vi "ordersCH3.vi"(8 "错误输入（无错误）":errorcluster, 9 "关闭通道":u16(ring)=1 items=["CH1", "CH2", "CH3", "CH4"], 10 "打开通道":u16(ring)=2 items=["CH1", "CH2", "CH3", "CH4"], 11 "VISA资源名称":refnum<visa-resource-name>="DPO5054-C012667") -> (0 "错误输出":errorcluster, 2 "输出数组":dbl[](array[numeric]))   [LabVIEW 2014]
panel:
  out "AMP":dbl
  out "RMS":dbl
  out "MAX":dbl
  out "MIN":dbl
  out "PK2PK":dbl
  out "PERIOD":dbl
  out "FREQ":dbl
  out "RISETIME":dbl
  out "FallTime":dbl
  out "PosWidth":dbl
  out "NegWidth":dbl
  out "PositiveDutyCycle":dbl
  out "NegativeDutyCycle":dbl
  out "ACRMS":dbl
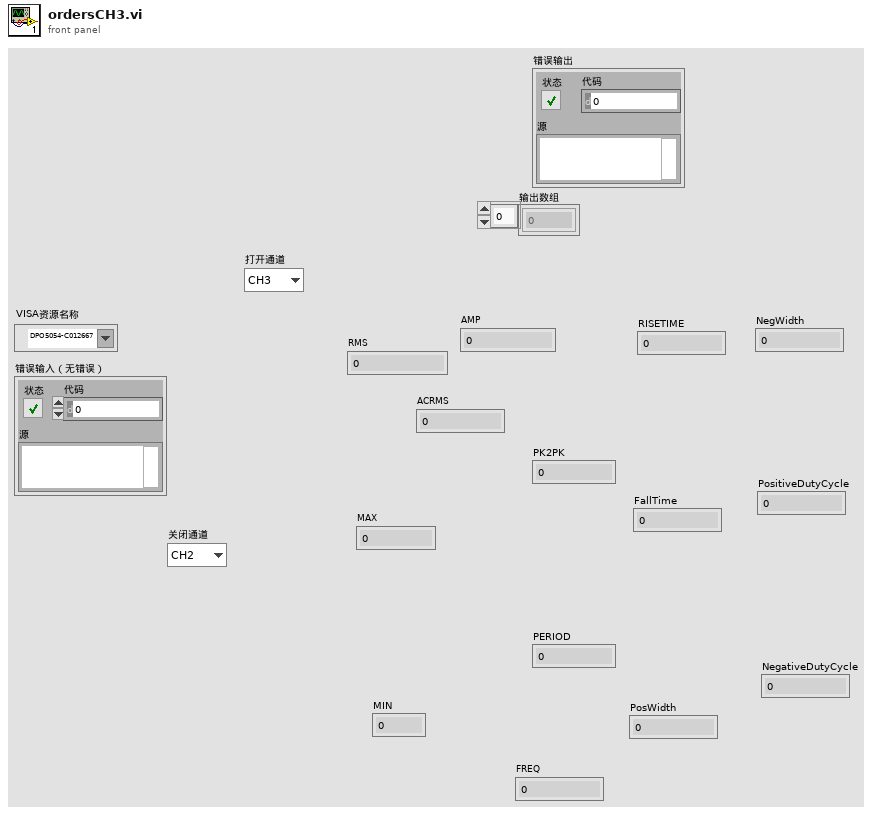
[diagram p1: front panel]
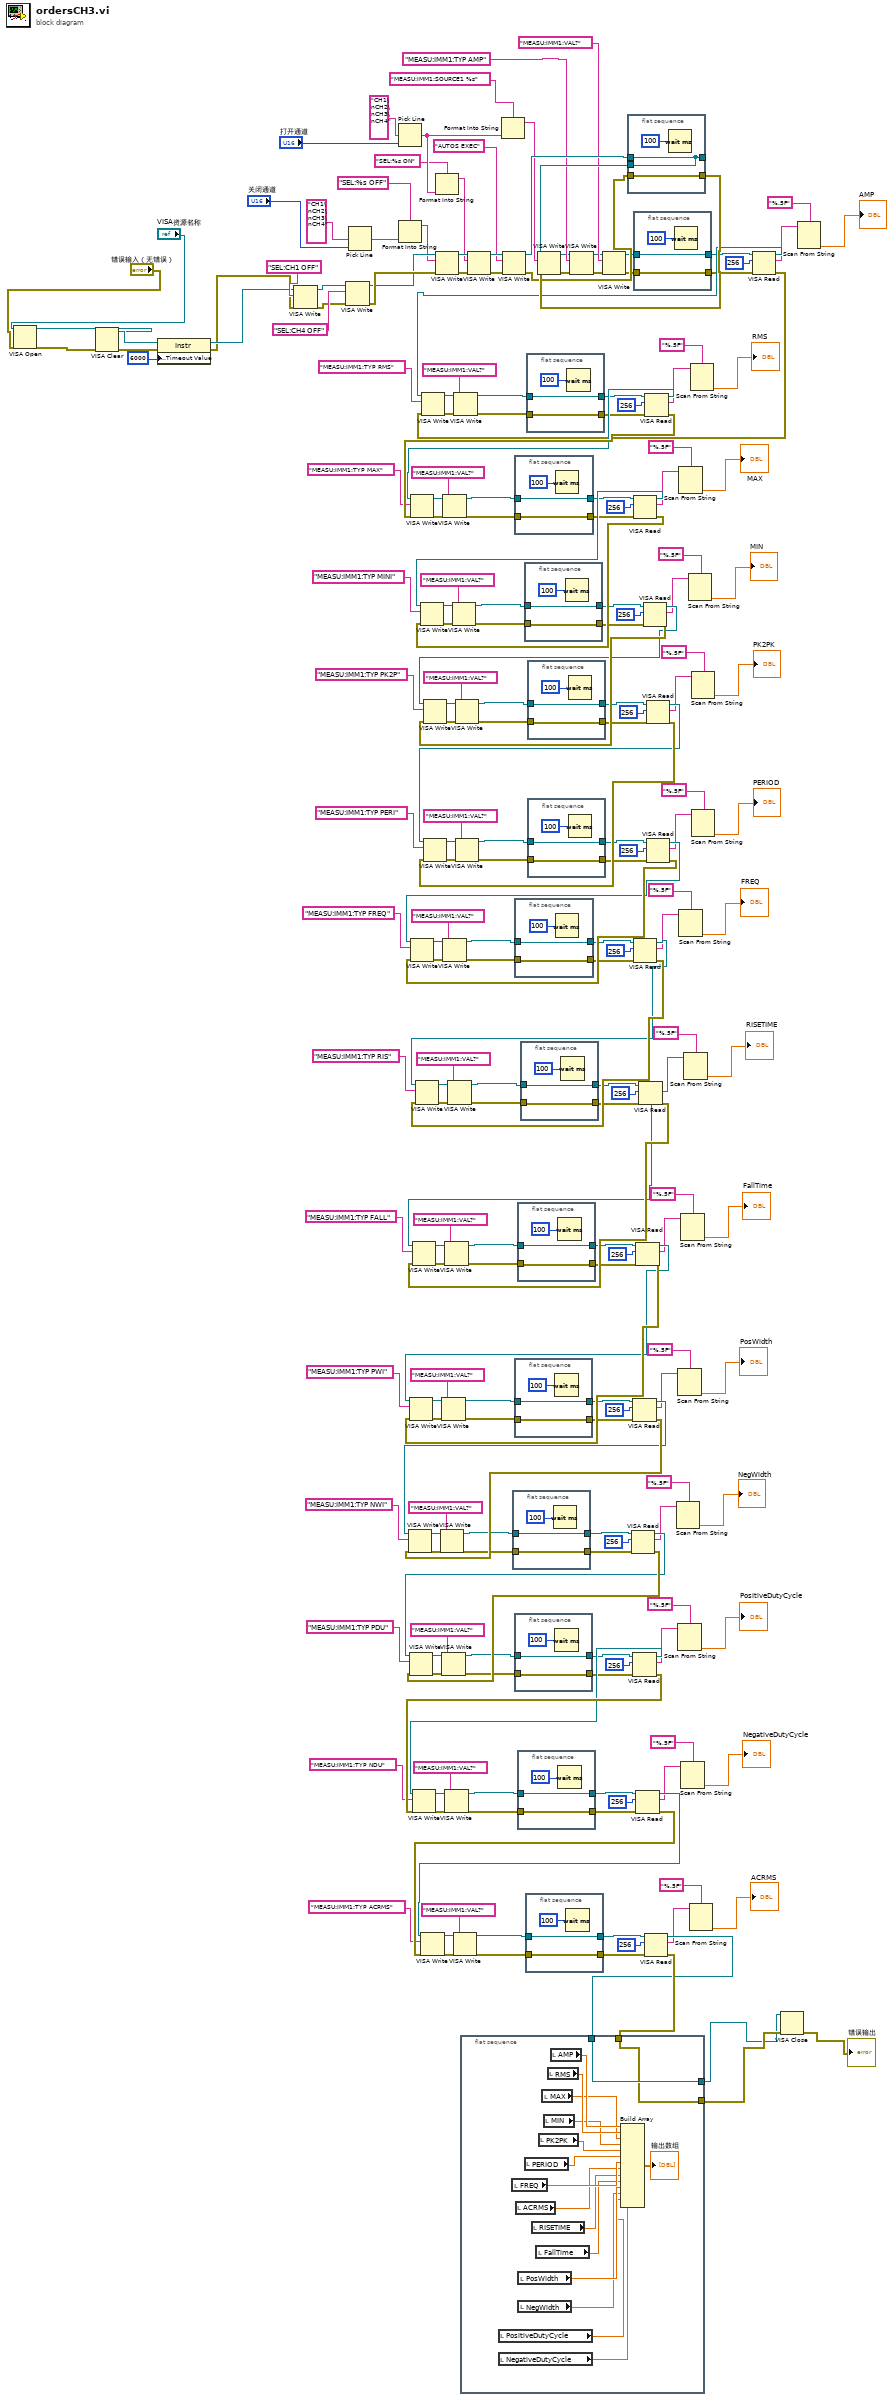
[diagram p0: block diagram]
diagram:
  n1 = VISA Open(error in (no error)="错误输入（无错误）", VISA resource name="VISA资源名称") -> (VISA resource name=w221:refnum<visa-resource-name>, error out=w222:errorcluster)  [unwired: 3 in]
  n2 = VISA Clear(VISA resource name=w221, error in (no error)=w222) -> (VISA resource name out=w223:refnum<visa-resource-name>, error out=w224:errorcluster)
  n3 = property class="Instr"(reference=w223, error in=w224, "General Settings:Timeout Value"=u32 6000) -> (reference out=w231:refnum<visa-resource-name>, error out=w230:errorcluster)
  n4 = VISA Write(VISA resource name=w231, write buffer="SEL:CH1 OFF" ("格式字符串"), error in (no error)=w230) -> (VISA resource name out=w233:refnum<visa-resource-name>, error out=w234:errorcluster)  [unwired: 1 out]
  n5 = VISA Write(VISA resource name=w233, write buffer="SEL:CH4 OFF" ("格式字符串"), error in (no error)=w234) -> (VISA resource name out=w236:refnum<visa-resource-name>, error out=w237:errorcluster)  [unwired: 1 out]
  n6 = Pick Line(multi-line string="CH1\nCH2\nCH3\nCH4" ("多行字符串"), line index="关闭通道") -> (output string=w21:string)  [unwired: 1 in]
  n7 = Pick Line(multi-line string="CH1\nCH2\nCH3\nCH4" ("多行字符串"), line index="打开通道") -> (output string=w16:string)  [unwired: 1 in]
  n8 = Format Into String(format string="SEL:%s OFF" ("格式字符串"), w21) -> (resulting string=w25:string)  [unwired: 2 in, 1 out]
  n9 = Format Into String(format string="SEL:%s ON" ("格式字符串"), w16) -> (resulting string=w17:string)  [unwired: 2 in, 1 out]
  n10 = VISA Write(VISA resource name=w236, write buffer=w25, error in (no error)=w237) -> (VISA resource name out=w26:refnum<visa-resource-name>, error out=w27:errorcluster)  [unwired: 1 out]
  n11 = flat-sequence {
    tunnel: w218 -> [w239]
    tunnel: [w239] -> w227
    tunnel: w219 -> [w238]
    tunnel: [w238] -> w228
    frame #0 {
      n12 = local read "PositiveDutyCycle"() -> (w242:dbl)
      n13 = local read "NegativeDutyCycle"() -> (w241:dbl)
      n14 = local read "FREQ"() -> (w248:dbl)
      n15 = local read "ACRMS"() -> (w247:dbl)
      n16 = local read "PosWidth"() -> (w244:dbl)
      n17 = local read "NegWidth"() -> (w243:dbl)
      n18 = local read "PERIOD"() -> (w249:dbl)
      n19 = local read "RISETIME"() -> (w246:dbl)
      n20 = local read "FallTime"() -> (w245:dbl)
      n21 = local read "PK2PK"() -> (w250:dbl)
      n22 = local read "MAX"() -> (w252:dbl)
      n23 = local read "MIN"() -> (w251:dbl)
      n24 = local read "RMS"() -> (w253:dbl)
      n25 = local read "AMP"() -> (w254:dbl)
      n26 = Build Array(w254, w253, w252, w251, w250, w249, w248, w247, w246, w245, w244, w243, w242, w241) -> (→"输出数组":dbl[])
    }
  }
  n27 = VISA Write(VISA resource name=w26, write buffer=w17, error in (no error)=w27) -> (VISA resource name out=w19:refnum<visa-resource-name>, error out=w20:errorcluster)  [unwired: 1 out]
  n28 = Format Into String(format string="MEASU:IMM1:SOURCE1 %s" ("格式字符串"), w16) -> (resulting string=w3:string)  [unwired: 2 in, 1 out]
  n29 = VISA Write(VISA resource name=w19, write buffer="AUTOS EXEC" ("写入缓冲区"), error in (no error)=w20) -> (VISA resource name out=w116:refnum<visa-resource-name>, error out=w117:errorcluster)  [unwired: 1 out]
  n30 = flat-sequence {
    tunnel: w157 -> [w256]
    tunnel: [w256] -> w159
    tunnel: w156 -> [w255]
    tunnel: [w255] -> w160
    frame #0 {
      n31 = Wait (ms)(milliseconds to wait=u32 100 ("等待时间（毫秒）")) -> ()  [unwired: 1 out]
    }
  }
  n32 = flat-sequence {
    tunnel: w154 -> [w259]
    tunnel: [w259] -> w152
    tunnel: w155 -> [w258]
    tunnel: [w258] -> w151
    frame #0 {
      n33 = Wait (ms)(milliseconds to wait=u32 100 ("等待时间（毫秒）")) -> ()  [unwired: 1 out]
    }
  }
  n34 = flat-sequence {
    tunnel: w178 -> [w262]
    tunnel: [w262] -> w176
    tunnel: w179 -> [w261]
    tunnel: [w261] -> w175
    frame #0 {
      n35 = Wait (ms)(milliseconds to wait=u32 100 ("等待时间（毫秒）")) -> ()  [unwired: 1 out]
    }
  }
  n36 = flat-sequence {
    tunnel: w45 -> [w265]
    tunnel: [w265] -> w47
    tunnel: w44 -> [w264]
    tunnel: [w264] -> w48
    frame #0 {
      n37 = Wait (ms)(milliseconds to wait=u32 100 ("等待时间（毫秒）")) -> ()  [unwired: 1 out]
    }
  }
  n38 = flat-sequence {
    tunnel: w93 -> [w268]
    tunnel: [w268] -> w95
    tunnel: w92 -> [w267]
    tunnel: [w267] -> w96
    frame #0 {
      n39 = Wait (ms)(milliseconds to wait=u32 100 ("等待时间（毫秒）")) -> ()  [unwired: 1 out]
    }
  }
  n40 = flat-sequence {
    tunnel: w133 -> [w271]
    tunnel: [w271] -> w135
    tunnel: w132 -> [w270]
    tunnel: [w270] -> w136
    frame #0 {
      n41 = Wait (ms)(milliseconds to wait=u32 100 ("等待时间（毫秒）")) -> ()  [unwired: 1 out]
    }
  }
  n42 = flat-sequence {
    tunnel: w181 -> [w274]
    tunnel: [w274] -> w183
    tunnel: w180 -> [w273]
    tunnel: [w273] -> w184
    frame #0 {
      n43 = Wait (ms)(milliseconds to wait=u32 100 ("等待时间（毫秒）")) -> ()  [unwired: 1 out]
    }
  }
  n44 = flat-sequence {
    tunnel: w130 -> [w277]
    tunnel: [w277] -> w128
    tunnel: w131 -> [w276]
    tunnel: [w276] -> w127
    frame #0 {
      n45 = Wait (ms)(milliseconds to wait=u32 100 ("等待时间（毫秒）")) -> ()  [unwired: 1 out]
    }
  }
  n46 = flat-sequence {
    tunnel: w66 -> [w280]
    tunnel: [w280] -> w64
    tunnel: w67 -> [w279]
    tunnel: [w279] -> w63
    frame #0 {
      n47 = Wait (ms)(milliseconds to wait=u32 100 ("等待时间（毫秒）")) -> ()  [unwired: 1 out]
    }
  }
  n48 = flat-sequence {
    tunnel: w214 -> [w283]
    tunnel: [w283] -> w212
    tunnel: w215 -> [w282]
    tunnel: [w282] -> w211
    frame #0 {
      n49 = Wait (ms)(milliseconds to wait=u32 100 ("等待时间（毫秒）")) -> ()  [unwired: 1 out]
    }
  }
  n50 = flat-sequence {
    tunnel: w42 -> [w286]
    tunnel: [w286] -> w40
    tunnel: w43 -> [w285]
    tunnel: [w285] -> w39
    frame #0 {
      n51 = Wait (ms)(milliseconds to wait=u32 100 ("等待时间（毫秒）")) -> ()  [unwired: 1 out]
    }
  }
  n52 = flat-sequence {
    tunnel: w69 -> [w289]
    tunnel: [w289] -> w71
    tunnel: w68 -> [w288]
    tunnel: [w288] -> w72
    frame #0 {
      n53 = Wait (ms)(milliseconds to wait=u32 100 ("等待时间（毫秒）")) -> ()  [unwired: 1 out]
    }
  }
  n54 = flat-sequence {
    tunnel: w90 -> [w292]
    tunnel: [w292] -> w88
    tunnel: w91 -> [w291]
    tunnel: [w291] -> w87
    frame #0 {
      n55 = Wait (ms)(milliseconds to wait=u32 100 ("等待时间（毫秒）")) -> ()  [unwired: 1 out]
    }
  }
  n56 = VISA Write(VISA resource name=w118, write buffer=w3, error in (no error)=w119) -> (VISA resource name out=w6:refnum<visa-resource-name>, error out=w7:errorcluster)  [unwired: 1 out]
  n57 = VISA Write(VISA resource name=w6, write buffer="MEASU:IMM1:TYP AMP" ("写入缓冲区"), error in (no error)=w7) -> (VISA resource name out=w10:refnum<visa-resource-name>, error out=w11:errorcluster)  [unwired: 1 out]
  n58 = VISA Write(VISA resource name=w10, write buffer="MEASU:IMM1:VAL?" ("写入缓冲区"), error in (no error)=w11) -> (VISA resource name out=w13:refnum<visa-resource-name>, error out=w14:errorcluster)  [unwired: 1 out]
  n59 = flat-sequence {
    tunnel: w116 -> [w294]
    tunnel: [w294] -> _
    tunnel: w117 -> [w295]
    tunnel: [w295] -> w119
    tunnel: [w294] -> w118
    frame #0 {
      n60 = Wait (ms)(milliseconds to wait=u32 100 ("等待时间（毫秒）")) -> ()  [unwired: 1 out]
    }
  }
  n61 = VISA Read(VISA resource name=w159, byte count=u32 256 ("字节总数"), error in (no error)=w160) -> (VISA resource name out=w200:refnum<visa-resource-name>, read buffer=w161:string, error out=w201:errorcluster)  [unwired: 1 out]
  n62 = VISA Write(VISA resource name=w200, write buffer="MEASU:IMM1:TYP PDU" ("写入缓冲区"), error in (no error)=w201) -> (VISA resource name out=w170:refnum<visa-resource-name>, error out=w169:errorcluster)  [unwired: 1 out]
  n63 = VISA Write(VISA resource name=w170, write buffer="MEASU:IMM1:VAL?" ("写入缓冲区"), error in (no error)=w169) -> (VISA resource name out=w178:refnum<visa-resource-name>, error out=w179:errorcluster)  [unwired: 1 out]
  n64 = VISA Read(VISA resource name=w152, byte count=u32 256 ("字节总数"), error in (no error)=w151) -> (VISA resource name out=w198:refnum<visa-resource-name>, read buffer=w150:string, error out=w199:errorcluster)  [unwired: 1 out]
  n65 = VISA Write(VISA resource name=w198, write buffer="MEASU:IMM1:TYP NWI" ("写入缓冲区"), error in (no error)=w199) -> (VISA resource name out=w165:refnum<visa-resource-name>, error out=w166:errorcluster)  [unwired: 1 out]
  n66 = VISA Write(VISA resource name=w165, write buffer="MEASU:IMM1:VAL?" ("写入缓冲区"), error in (no error)=w166) -> (VISA resource name out=w157:refnum<visa-resource-name>, error out=w156:errorcluster)  [unwired: 1 out]
  n67 = VISA Read(VISA resource name=w176, byte count=u32 256 ("字节总数"), error in (no error)=w175) -> (VISA resource name out=w202:refnum<visa-resource-name>, read buffer=w174:string, error out=w203:errorcluster)  [unwired: 1 out]
  n68 = VISA Write(VISA resource name=w202, write buffer="MEASU:IMM1:TYP NDU" ("写入缓冲区"), error in (no error)=w203) -> (VISA resource name out=w189:refnum<visa-resource-name>, error out=w190:errorcluster)  [unwired: 1 out]
  n69 = VISA Write(VISA resource name=w189, write buffer="MEASU:IMM1:VAL?" ("写入缓冲区"), error in (no error)=w190) -> (VISA resource name out=w181:refnum<visa-resource-name>, error out=w180:errorcluster)  [unwired: 1 out]
  n70 = flat-sequence {
    tunnel: w13 -> [w298]
    tunnel: [w298] -> w8
    tunnel: w14 -> [w297]
    tunnel: [w297] -> w9
    frame #0 {
      n71 = Wait (ms)(milliseconds to wait=u32 100 ("等待时间（毫秒）")) -> ()  [unwired: 1 out]
    }
  }
  n72 = VISA Read(VISA resource name=w47, byte count=u32 256 ("字节总数"), error in (no error)=w48) -> (VISA resource name out=w108:refnum<visa-resource-name>, read buffer=w49:string, error out=w109:errorcluster)  [unwired: 1 out]
  n73 = VISA Write(VISA resource name=w108, write buffer="MEASU:IMM1:TYP MINI" ("写入缓冲区"), error in (no error)=w109) -> (VISA resource name out=w58:refnum<visa-resource-name>, error out=w57:errorcluster)  [unwired: 1 out]
  n74 = VISA Write(VISA resource name=w58, write buffer="MEASU:IMM1:VAL?" ("写入缓冲区"), error in (no error)=w57) -> (VISA resource name out=w66:refnum<visa-resource-name>, error out=w67:errorcluster)  [unwired: 1 out]
  n75 = VISA Read(VISA resource name=w95, byte count=u32 256 ("字节总数"), error in (no error)=w96) -> (VISA resource name out=w192:refnum<visa-resource-name>, read buffer=w97:string, error out=w193:errorcluster)  [unwired: 1 out]
  n76 = VISA Write(VISA resource name=w192, write buffer="MEASU:IMM1:TYP RIS" ("写入缓冲区"), error in (no error)=w193) -> (VISA resource name out=w122:refnum<visa-resource-name>, error out=w121:errorcluster)  [unwired: 1 out]
  n77 = VISA Write(VISA resource name=w122, write buffer="MEASU:IMM1:VAL?" ("写入缓冲区"), error in (no error)=w121) -> (VISA resource name out=w130:refnum<visa-resource-name>, error out=w131:errorcluster)  [unwired: 1 out]
  n78 = VISA Read(VISA resource name=w135, byte count=u32 256 ("字节总数"), error in (no error)=w136) -> (VISA resource name out=w196:refnum<visa-resource-name>, read buffer=w137:string, error out=w197:errorcluster)  [unwired: 1 out]
  n79 = VISA Write(VISA resource name=w196, write buffer="MEASU:IMM1:TYP PWI" ("写入缓冲区"), error in (no error)=w197) -> (VISA resource name out=w146:refnum<visa-resource-name>, error out=w145:errorcluster)  [unwired: 1 out]
  n80 = VISA Write(VISA resource name=w146, write buffer="MEASU:IMM1:VAL?" ("写入缓冲区"), error in (no error)=w145) -> (VISA resource name out=w154:refnum<visa-resource-name>, error out=w155:errorcluster)  [unwired: 1 out]
  n81 = VISA Read(VISA resource name=w183, byte count=u32 256 ("字节总数"), error in (no error)=w184) -> (VISA resource name out=w216:refnum<visa-resource-name>, read buffer=w185:string, error out=w217:errorcluster)  [unwired: 1 out]
  n82 = VISA Write(VISA resource name=w216, write buffer="MEASU:IMM1:TYP ACRMS" ("写入缓冲区"), error in (no error)=w217) -> (VISA resource name out=w206:refnum<visa-resource-name>, error out=w205:errorcluster)  [unwired: 1 out]
  n83 = VISA Write(VISA resource name=w206, write buffer="MEASU:IMM1:VAL?" ("写入缓冲区"), error in (no error)=w205) -> (VISA resource name out=w214:refnum<visa-resource-name>, error out=w215:errorcluster)  [unwired: 1 out]
  n84 = VISA Read(VISA resource name=w128, byte count=u32 256 ("字节总数"), error in (no error)=w127) -> (VISA resource name out=w194:refnum<visa-resource-name>, read buffer=w126:string, error out=w195:errorcluster)  [unwired: 1 out]
  n85 = VISA Write(VISA resource name=w194, write buffer="MEASU:IMM1:TYP FALL" ("写入缓冲区"), error in (no error)=w195) -> (VISA resource name out=w141:refnum<visa-resource-name>, error out=w142:errorcluster)  [unwired: 1 out]
  n86 = VISA Write(VISA resource name=w141, write buffer="MEASU:IMM1:VAL?" ("写入缓冲区"), error in (no error)=w142) -> (VISA resource name out=w133:refnum<visa-resource-name>, error out=w132:errorcluster)  [unwired: 1 out]
  n87 = VISA Read(VISA resource name=w64, byte count=u32 256 ("字节总数"), error in (no error)=w63) -> (VISA resource name out=w110:refnum<visa-resource-name>, read buffer=w62:string, error out=w111:errorcluster)  [unwired: 1 out]
  n88 = VISA Write(VISA resource name=w110, write buffer="MEASU:IMM1:TYP PK2P" ("写入缓冲区"), error in (no error)=w111) -> (VISA resource name out=w77:refnum<visa-resource-name>, error out=w78:errorcluster)  [unwired: 1 out]
  n89 = VISA Write(VISA resource name=w77, write buffer="MEASU:IMM1:VAL?" ("写入缓冲区"), error in (no error)=w78) -> (VISA resource name out=w69:refnum<visa-resource-name>, error out=w68:errorcluster)  [unwired: 1 out]
  n90 = VISA Read(VISA resource name=w212, byte count=u32 256 ("字节总数"), error in (no error)=w211) -> (VISA resource name out=w218:refnum<visa-resource-name>, read buffer=w210:string, error out=w219:errorcluster)  [unwired: 1 out]
  n91 = VISA Read(VISA resource name=w40, byte count=u32 256 ("字节总数"), error in (no error)=w39) -> (VISA resource name out=w106:refnum<visa-resource-name>, read buffer=w38:string, error out=w107:errorcluster)  [unwired: 1 out]
  n92 = VISA Write(VISA resource name=w106, write buffer="MEASU:IMM1:TYP MAX" ("写入缓冲区"), error in (no error)=w107) -> (VISA resource name out=w53:refnum<visa-resource-name>, error out=w54:errorcluster)  [unwired: 1 out]
  n93 = VISA Write(VISA resource name=w53, write buffer="MEASU:IMM1:VAL?" ("写入缓冲区"), error in (no error)=w54) -> (VISA resource name out=w45:refnum<visa-resource-name>, error out=w44:errorcluster)  [unwired: 1 out]
  n94 = VISA Read(VISA resource name=w71, byte count=u32 256 ("字节总数"), error in (no error)=w72) -> (VISA resource name out=w112:refnum<visa-resource-name>, read buffer=w73:string, error out=w113:errorcluster)  [unwired: 1 out]
  n95 = VISA Write(VISA resource name=w112, write buffer="MEASU:IMM1:TYP PERI" ("写入缓冲区"), error in (no error)=w113) -> (VISA resource name out=w82:refnum<visa-resource-name>, error out=w81:errorcluster)  [unwired: 1 out]
  n96 = VISA Write(VISA resource name=w82, write buffer="MEASU:IMM1:VAL?" ("写入缓冲区"), error in (no error)=w81) -> (VISA resource name out=w90:refnum<visa-resource-name>, error out=w91:errorcluster)  [unwired: 1 out]
  n97 = VISA Read(VISA resource name=w88, byte count=u32 256 ("字节总数"), error in (no error)=w87) -> (VISA resource name out=w114:refnum<visa-resource-name>, read buffer=w86:string, error out=w115:errorcluster)  [unwired: 1 out]
  n98 = VISA Write(VISA resource name=w114, write buffer="MEASU:IMM1:TYP FREQ" ("写入缓冲区"), error in (no error)=w115) -> (VISA resource name out=w101:refnum<visa-resource-name>, error out=w102:errorcluster)  [unwired: 1 out]
  n99 = VISA Write(VISA resource name=w101, write buffer="MEASU:IMM1:VAL?" ("写入缓冲区"), error in (no error)=w102) -> (VISA resource name out=w93:refnum<visa-resource-name>, error out=w92:errorcluster)  [unwired: 1 out]
  n100 = Scan From String(format string="%.5F" ("格式字符串"), input string=w161) -> (output 1=→"NegWidth":dbl)  [unwired: 3 in, 3 out]
  n101 = Scan From String(format string="%.5F" ("格式字符串"), input string=w150) -> (output 1=→"PosWidth":dbl)  [unwired: 3 in, 3 out]
  n102 = Scan From String(format string="%.5F" ("格式字符串"), input string=w174) -> (output 1=→"PositiveDutyCycle":dbl)  [unwired: 3 in, 3 out]
  n103 = Scan From String(format string="%.5F" ("格式字符串"), input string=w49) -> (output 1=→"MAX":dbl)  [unwired: 3 in, 3 out]
  n104 = Scan From String(format string="%.5F" ("格式字符串"), input string=w97) -> (output 1=→"FREQ":dbl)  [unwired: 3 in, 3 out]
  n105 = Scan From String(format string="%.5F" ("格式字符串"), input string=w137) -> (output 1=→"FallTime":dbl)  [unwired: 3 in, 3 out]
  n106 = Scan From String(format string="%.5F" ("格式字符串"), input string=w185) -> (output 1=→"NegativeDutyCycle":dbl)  [unwired: 3 in, 3 out]
  n107 = Scan From String(format string="%.5F" ("格式字符串"), input string=w126) -> (output 1=→"RISETIME":dbl)  [unwired: 3 in, 3 out]
  n108 = Scan From String(format string="%.5F" ("格式字符串"), input string=w62) -> (output 1=→"MIN":dbl)  [unwired: 3 in, 3 out]
  n109 = Scan From String(format string="%.5F" ("格式字符串"), input string=w210) -> (output 1=→"ACRMS":dbl)  [unwired: 3 in, 3 out]
  n110 = Scan From String(format string="%.5F" ("格式字符串"), input string=w38) -> (output 1=→"RMS":dbl)  [unwired: 3 in, 3 out]
  n111 = Scan From String(format string="%.5F" ("格式字符串"), input string=w73) -> (output 1=→"PK2PK":dbl)  [unwired: 3 in, 3 out]
  n112 = Scan From String(format string="%.5F" ("格式字符串"), input string=w86) -> (output 1=→"PERIOD":dbl)  [unwired: 3 in, 3 out]
  n113 = VISA Read(VISA resource name=w8, byte count=u32 256 ("字节总数"), error in (no error)=w9) -> (VISA resource name out=w104:refnum<visa-resource-name>, read buffer=w29:string, error out=w105:errorcluster)  [unwired: 1 out]
  n114 = VISA Write(VISA resource name=w104, write buffer="MEASU:IMM1:TYP RMS" ("写入缓冲区"), error in (no error)=w105) -> (VISA resource name out=w34:refnum<visa-resource-name>, error out=w33:errorcluster)  [unwired: 1 out]
  n115 = VISA Write(VISA resource name=w34, write buffer="MEASU:IMM1:VAL?" ("写入缓冲区"), error in (no error)=w33) -> (VISA resource name out=w42:refnum<visa-resource-name>, error out=w43:errorcluster)  [unwired: 1 out]
  n116 = VISA Close(VISA resource name=w227, error in (no error)=w228) -> (error out=→"错误输出":errorcluster)
  n117 = Scan From String(format string="%.5F" ("格式字符串"), input string=w29) -> (output 1=→"AMP":dbl)  [unwired: 3 in, 3 out]
